vi "Incorrect Tag String Error.vi"(8 "error in (no error)":errorcluster, 11 "Tag":string) -> (0 "error out":errorcluster)   [LabVIEW 2021, in "Var Bus.lvclass"]
uses:
  Var Bus.lvclass
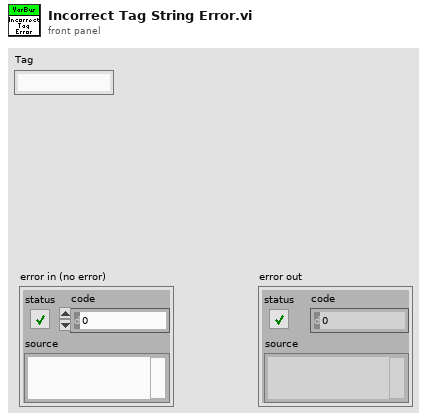
[diagram p1: front panel]
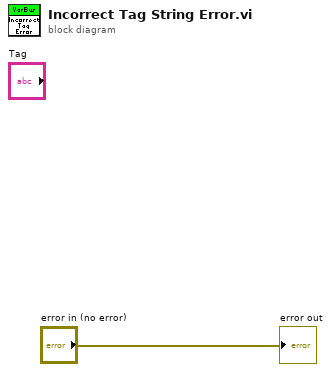
[diagram p0: block diagram]
diagram:
  "error out" <- "error in (no error)"
